vi "SortRobotsById.vi"(0 "object in":refnum<class "DefendAreaTactic.lvclass">, 2 "robots in":refnum<class "Robot.lvclass">[](array[class]), 5 "error in (no error)":errorcluster) -> (14 "object out":refnum<class "DefendAreaTactic.lvclass">, 16 "robots out":refnum<class "Robot.lvclass">[](array[class]), 19 "error out":errorcluster)   [LabVIEW 2024, in "DefendAreaTactic.lvclass"]
uses:
  DefendAreaTactic.lvclass
  Robot_class/Robot.lvclass
  Robot_class/Robot.lvclass/Robot.ctl
  Robot_class/Read id.vi
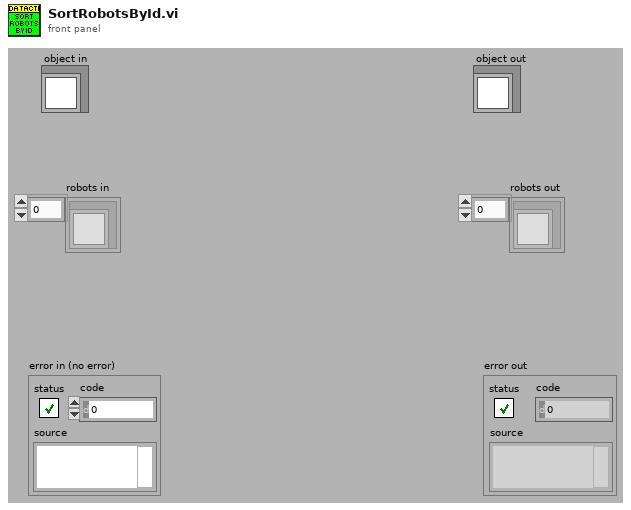
[diagram p1: front panel]
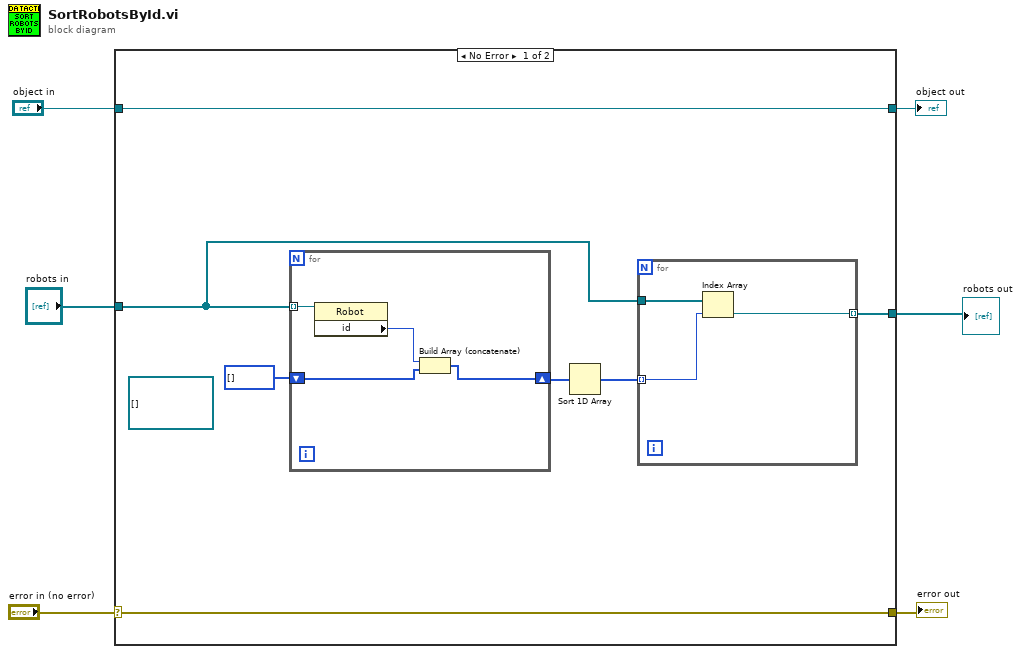
[diagram p0: block diagram]
diagram:
  n1 = case shown="No Error" "error in (no error)" {
    selector: "error in (no error)" -> [w13 w23]
    tunnel: [w13 w23] -> w5
    tunnel: [w12 w22] -> w3
    tunnel: "object in" -> [w12 w22]
    tunnel: "robots in" -> [w9 w21]
    tunnel: [w7 w21] -> w1
    frame No Error {
      (unwired) refnum<class "Robot.lvclass">[] [] ("Array")
      n2 = for {
        tunnel: w9 -> [w20] mode=indexing
        shift-right: [w17] -> w10
        shift-left: i32[] [] -> [w18]
        n3 = property class="Robot"(reference=w20) -> ("id"=w19:i32)  [unwired: 1 in, 2 out]
        n4 = Build Array (concatenate)(w19, w18) -> (w17:i32[])
      }
      n5 = Sort 1D Array(array=w10) -> (sorted array=w8:i32[])
      n6 = for {
        tunnel: w9 -> [w16]
        tunnel: w8 -> [w15] mode=indexing
        tunnel: [w14] -> w7 mode=indexing
        n7 = Index Array(array=w16, index=w15) -> (element=w14:refnum<class "Robot.lvclass">)
      }
    }
    frame Error {
    }
  }
  "error out" <- w5
  "object out" <- w3
  "robots out" <- w1
